vi "Save DAC Configuration.vi"(8 "error in":errorcluster, 10 "Config File refnum in":T1, 11 "DAC Keller Diff P 23X in":refnum<class "DAC Keller Diff P 23X.lvclass">) -> (0 "error out":errorcluster, 2 "Config File refnum out":T1, 3 "DAC Keller Diff P 23X out":refnum<class "DAC Keller Diff P 23X.lvclass">)   [LabVIEW 2019, in "DAC.lvlib" / "DAC Keller Diff P 23X.lvclass"]
uses:
  DAC Keller Diff P 23X.lvclass
  C:/Users/krio/Documents/LV_Projects/test-stand/App/DAC/DAC.lvclass
  <vilib>/Utility/config.llb/Config Data RefNum.ctl
  DAC.lvclass/DAC.ctl
  DAC Keller Diff P 23X.lvclass/DAC Keller Diff P 23X.ctl
  <vilib>/Utility/config.llb/Write Key (String).vi
  DAC.lvclass
  <vilib>/Utility/config.llb/NI_LVConfig.lvlib
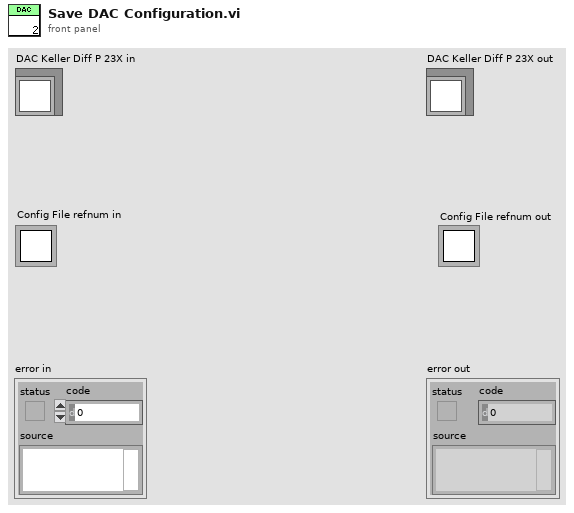
[diagram p1: front panel]
types:
  T1 = typedef "NI_LVConfig.lvlib/Config Data RefNum.ctl" = refnum<k1>
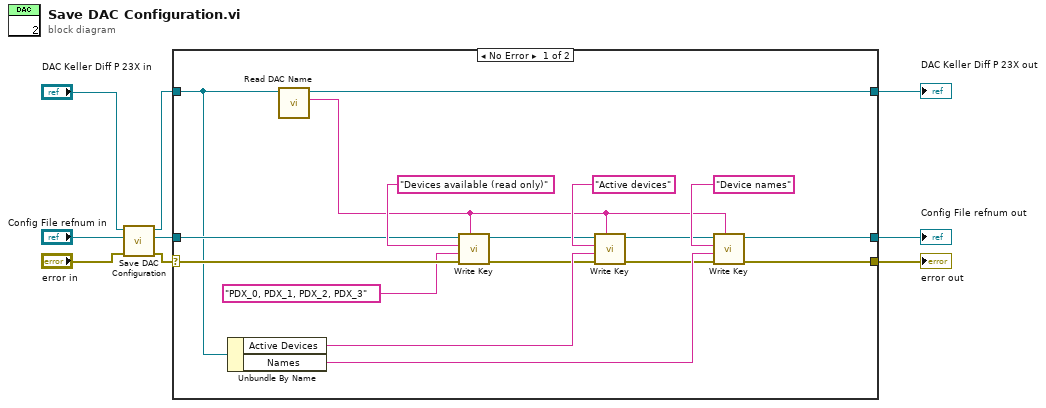
[diagram p0: block diagram]
diagram:
  n1 = call-parent "Save DAC Configuration.vi"("error in"="error in", "Config File refnum in"="Config File refnum in", "DAC in"="DAC Keller Diff P 23X in") -> ("error out"=w4:errorcluster, "Config File refnum out"=w5:T1, "DAC out"=w6:refnum<class "DAC Keller Diff P 23X.lvclass">)  [unwired: 6 in]
  n2 = case shown="No Error" w4 {
    selector: w4 -> [w24 w29]
    tunnel: [w11 w29] -> w1
    tunnel: [w22 w28] -> w3
    tunnel: w6 -> [w23 w28]
    tunnel: w5 -> [w25 w27]
    tunnel: [w14 w27] -> w2
    frame No Error {
      n3 = Unbundle By Name(w23) -> ("Active Devices"=w18:string, "Names"=w17:string)
      n4 = call "Read DAC Name.vi"("DAC in"=w23) -> ("DAC Name"=w19:string, "DAC out"=w22:refnum<class "DAC Keller Diff P 23X.lvclass">)  [unwired: 8 in, 1 out]
      n5 = call-poly <vilib>:"Write Key.vi"("section"=w19, "error in (no error)"=w24, "value"="PDX_0, PDX_1, PDX_2, PDX_3", "key"="Devices available (read only)", "refnum"=w25) -> ("error out"=w13:errorcluster, "refnum out"=w16:T1)  [unwired: 4 in, 1 out]
      n6 = call-poly <vilib>:"Write Key.vi"("section"=w19, "error in (no error)"=w13, "value"=w18, "key"="Active devices", "refnum"=w16) -> ("error out"=w12:errorcluster, "refnum out"=w15:T1)  [unwired: 4 in, 1 out]
      n7 = call-poly <vilib>:"Write Key.vi"("section"=w19, "error in (no error)"=w12, "value"=w17, "key"="Device names", "refnum"=w15) -> ("error out"=w11:errorcluster, "refnum out"=w14:T1)  [unwired: 4 in, 1 out]
    }
    frame Error {
    }
  }
  "error out" <- w1
  "DAC Keller Diff P 23X out" <- w3
  "Config File refnum out" <- w2
